vi "Construct.vi"(1 "Color":u32(colorbox), 2 "Radius":i16) -> (0 "CircleShape out":refnum<class "CircleShape.lvclass">)   [LabVIEW 2022 SP3, in "CircleShape.lvclass"]
uses:
  CircleShape.lvclass
  CircleShape.lvclass/CircleShape.ctl
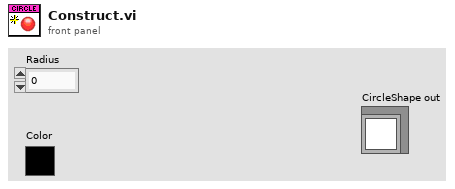
[diagram p1: front panel]
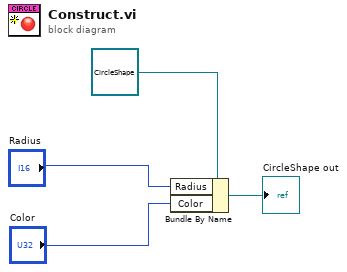
[diagram p0: block diagram]
diagram:
  n1 = Bundle By Name(cluster=refnum<class "CircleShape.lvclass"> refnum ("CircleShape.lvclass"), "Radius"="Radius", "Color"="Color") -> (→"CircleShape out":refnum<class "CircleShape.lvclass">)
